vi "Insert Into Array (Value).vi"(8 "error in (no error)":errorcluster, 9 "index":i32, 10 "JSON Value in":refnum<class "JSON Value.lvclass">, 11 "JSON Value in":refnum<class "JSON Value.lvclass">) -> (0 "error out":errorcluster, 3 "JSON Value out":refnum<class "JSON Value.lvclass">)   [LabVIEW 2017, in "JSON Value.lvclass"]
doc: "Inserts an element or subarray into a JSON array at the point you specify in index."
uses:
  JSON Value.lvclass
  JSON Value.lvclass/JSON Value.ctl
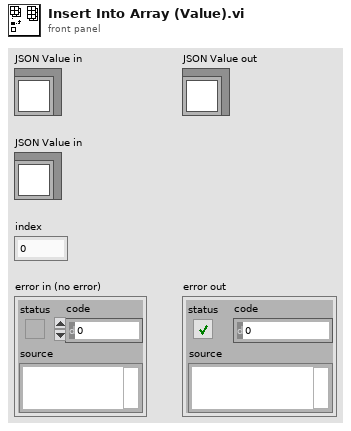
[diagram p1: front panel]
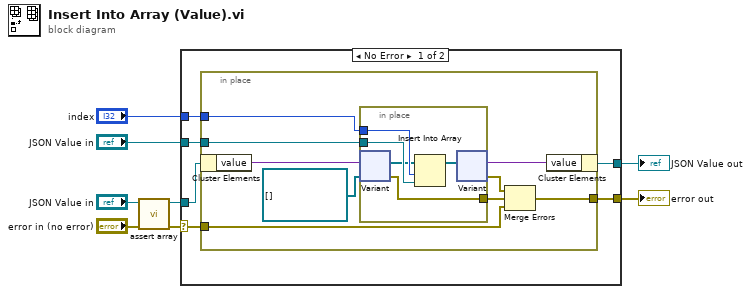
[diagram p0: block diagram]
diagram:
  n1 = call "assert array.vi"("error in (no error)"="error in (no error)", "JSON Value in"="JSON Value in") -> ("error out"=w2:errorcluster, "JSON Value out"=w4:refnum<class "JSON Value.lvclass">)  [unwired: 8 in]
  n2 = case shown="No Error" w2 {
    selector: w2 -> [w10 _]
    tunnel: [w14 w29] -> w7
    tunnel: "index" -> [w13 _]
    tunnel: "JSON Value in" -> [w12 w29]
    tunnel: w4 -> [w11 _]
    tunnel: [w9 _] -> w1
    frame No Error {
      n3 = in-place {
        in-place-border: w12 -> [w22]
        in-place-border: w13 -> [w23]
        in-place-border: w10 -> [w16]
        in-place-border: [w15] -> w9
        n4 = in-place-cluster #1(w11) -> ("value"=w21:variant)
        n5 = in-place {
          in-place-border: w23 -> [w28]
          in-place-border: w22 -> [w27]
          in-place-border: [w24] -> w17
          n6 = in-place-variant #2(w21, refnum<class "JSON Value.lvclass">[] [] ("output array")) -> (w26:refnum<class "JSON Value.lvclass">[], w24:errorcluster)
          n7 = Insert Into Array(array=w26, index=w28, new element=w27) -> (w25:refnum<class "JSON Value.lvclass">[])
          n8 = in-place-variant #2(w25) -> (w19:variant, w18:errorcluster)
        }
        n9 = Merge Errors(w18, w17, w16) -> (w15:errorcluster)
        n10 = in-place-cluster #1("value"=w19) -> (w14:refnum<class "JSON Value.lvclass">)
      }
    }
    frame Error {
    }
  }
  "JSON Value out" <- w7
  "error out" <- w1
